vi "Arduino_sendstring_test.vi"() -> ()   [LabVIEW 2015]
uses:
  <vilib>/Instr/_visa.llb/VISA Open Access Mode.ctl
  <vilib>/Instr/_visa.llb/VISA Configure Serial Port (Instr).vi
panel:
  out "Recived?":string
  in  "stop":bool
  in  "VISA resource name":refnum<visa-resource-name>
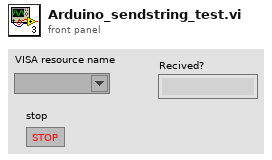
[diagram p1: front panel]
types:
  T1 = typedef "VISA Open Access Mode.ctl" = u32
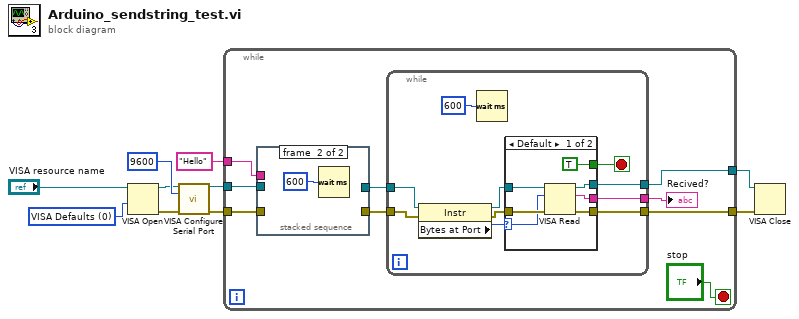
[diagram p0: block diagram]
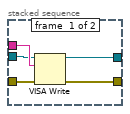
[diagram p2: hidden frame]
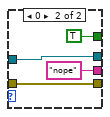
[diagram p3: hidden frame]
diagram:
  w4 = T1 0 items=["VISA Defaults"=0, "Exclusive Lock"=1, "Load Configured Settings"=4] ("Access Mode")
  n1 = VISA Open(access mode=w4, VISA resource name="VISA resource name") -> (VISA resource name=w6:refnum<visa-resource-name>, error out=w5:errorcluster)  [unwired: 3 in]
  n2 = call-poly "VISA Configure Serial Port"("VISA resource name"=w6, "baud rate (9600)"=u32 9600, "error in (no error)"=w5) -> ("VISA resource name out"=w9:refnum<visa-resource-name>, "error out"=w8:errorcluster)  [unwired: 11 in]
  n3 = while {
    tunnel: w9 -> [w14]
    tunnel: w8 -> [w13]
    tunnel: [w18] -> w3
    tunnel: [w17] -> w2
    tunnel: "Hello" -> [w15]
    stop <- "stop" stop-if-true
    n4 = stacked-sequence {
      tunnel: w15 -> [w24 _]
      tunnel: w14 -> [w23 _]
      tunnel: w13 -> [w22 _]
      tunnel: [w21 _] -> w12
      tunnel: [w20 _] -> w11
      frame #0 {
        n5 = VISA Write(VISA resource name=w23, write buffer=w24, error in (no error)=w22) -> (VISA resource name out=w21:refnum<visa-resource-name>, error out=w20:errorcluster)  [unwired: 1 out]
      }
      frame #1 {
        n6 = Wait (ms)(milliseconds to wait=u32 600) -> ()  [unwired: 1 out]
      }
    }
    n7 = while {
      tunnel: [w33] -> w18
      tunnel: [w32] -> w17
      tunnel: [w31] -> w16
      tunnel: w12 -> [w27]
      tunnel: w11 -> [w26]
      stop <- w34 stop-if-true
      n8 = property class="Instr"(reference=w27, error in=w26) -> (reference out=w29:refnum<visa-resource-name>, error out=w35:errorcluster, "Bytes at Port"=w30:u32)
      n9 = Wait (ms)(milliseconds to wait=u32 600) -> ()  [unwired: 1 out]
      n10 = case shown="Default" w30 {
        selector: w30 -> [w37 _]
        tunnel: w29 -> [w42 w46]
        tunnel: w35 -> [w41 w45]
        tunnel: [TRUE TRUE] -> w34
        tunnel: [w39 w45] -> w33
        tunnel: [w38 w46] -> w32
        tunnel: [w36 "nope"] -> w31
        frame Default {
          n11 = VISA Read(VISA resource name=w42, byte count=w37, error in (no error)=w41) -> (VISA resource name out=w38:refnum<visa-resource-name>, read buffer=w36:string, error out=w39:errorcluster)  [unwired: 1 out]
        }
        frame 0 {
        }
      }
    }
    "Recived?" <- w16
  }
  n12 = VISA Close(VISA resource name=w2, error in (no error)=w3) -> ()  [unwired: 1 out]
